vi "Get All Control Classes in Project.vi"() -> (3 "All Control Classes":refnum<vi>[](array[refnum]))   [LabVIEW 2015]
uses:
  Project Manipulation Scripts/Project Manipulation Scripts.lvlib
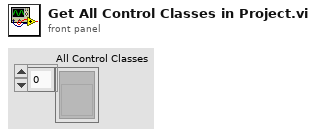
[diagram p1: front panel]
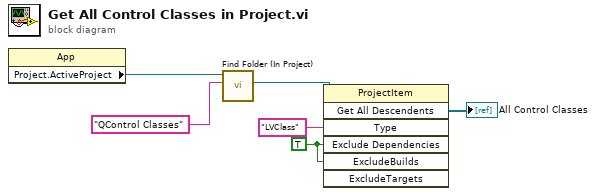
[diagram p0: block diagram]
diagram:
  w4 = TRUE ("ExcludeDependencies")
  n1 = property class="App"() -> ("Project.ActiveProject"=w2:refnum<vi>)  [unwired: 2 in, 2 out]
  n2 = call "Find Folder (In Project).vi"("Folder Name"="QControl Classes", "Project in"=w2) -> ("Folder Refnum"=w5:refnum<vi>)  [unwired: 7 in, 2 out]
  n3 = invoke class="ProjectItem" method="Get All Descendents"(reference=w5, "Type"="LVClass", "Exclude Dependencies"=w4, "ExcludeBuilds"=w4) -> ("All Descendents"=→"All Control Classes":refnum<vi>[])  [unwired: 3 in, 6 out]
